vi "domeADB_getResponse_VelocityMove.vi"(8 "error in (no error)":errorcluster, 11 "ackcmd_Ctl":T1={"cmdSeqNum"=0, "ack"=0, "error"=0, "result"="                                                                                                                                                                                                                                                                "}) -> (0 "error out":errorcluster, 2 "function return":i32, 3 "ackcmd_Ctl out":T1={"cmdSeqNum"=0, "ack"=0, "error"=0, "result"="                                                                                                                                                                                                                                                                "})   [LabVIEW 2016, in "SALLV_domeADB.lvlib"]
doc: "int domeADB_shm_getResponse_VelocityMoveLV(domeADB_ackcmdLV *ackcmd_Ctl);"
uses:
  SALLV_domeADB.lvlib
  DataTypes/ackcmd.ctl
  SALLV_domeADB.so
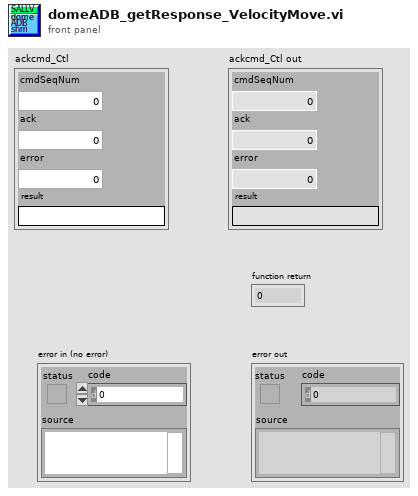
[diagram p1: front panel]
types:
  T1 = typedef "SALLV_domeADB.lvlib/ackcmd.ctl" = cluster{"cmdSeqNum":i32, "ack":i32, "error":i32, "result":string}
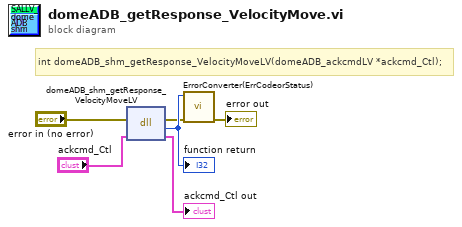
[diagram p0: block diagram]
diagram:
  # "int domeADB_shm_getResponse_VelocityMoveLV(domeADB_ackcmdLV *ackcmd_Ctl);"
  n1 = dll-call lib="home/andres/Desktop/SALLV_domeADB/SALLV_domeADB.*" fn="domeADB_shm_getResponse_VelocityMoveLV"(error in="error in (no error)", "ackcmd_Ctl"="ackcmd_Ctl") -> (error out=w2:errorcluster, w6:i32, "ackcmd_Ctl"=→"ackcmd_Ctl out":T1)  [unwired: 2 in, 1 out]
  "function return" <- w6
  n2 = call "ErrorConverter(ErrCodeorStatus).vi"("error in (no error)"=w2, "error code"=w6) -> ("error out"=→"error out":errorcluster)  [unwired: 9 in]
